vi "RND Integer.vi"(8 "Min":i32=1, 9 "Max":i32=9) -> (1 "RND Integer":i32)   [LabVIEW 2015, in "TSP Library.lvlib"]
uses:
  TSP Library.lvlib
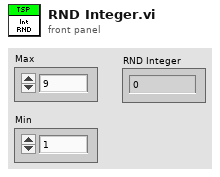
[diagram p1: front panel]
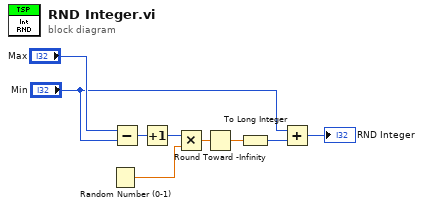
[diagram p0: block diagram]
diagram:
  n1 = Random Number (0-1)() -> (number: 0 to 1=w7:dbl)
  n2 = Subtract(x="Max", y="Min") -> (x-y=w8:i32)
  n3 = Increment(x=w8) -> (x+1=w2:i32)
  n4 = Multiply(x=w2, y=w7) -> (x*y=w6:dbl)
  n5 = Round Toward -Infinity(1:w6) -> (0:w1:dbl)
  n6 = To Long Integer(number=w1) -> (32bit integer=w4:i32)
  n7 = Add(x="Min", y=w4) -> (x+y=→"RND Integer":i32)
